vi "Autonomous Independent.vi"   [LabVIEW 2013]
doc: "This VI is called when autonomous begins, and will automatically be terminated when autonomous ends. You can carry out timed or sensor driven robot movement independently without needing to return to the caller."
uses:
  <vilib>/Rock Robotics/WPI/Solenoid/WPI_SolenoidValue.ctl
  Robot Global Data.vi
  <vilib>/Rock Robotics/WPI/RobotDrive/WPI_RobotDriveGetSetRefNum.vi
  <vilib>/Rock Robotics/WPI/RobotDrive/WPI_RobotDriveArcadeDrive_Standard(NoSaturation).vi
  <vilib>/Rock Robotics/WPI/Solenoid/Deprecated/WPI_SolenoidGetBool.vi
  <vilib>/Rock Robotics/WPI/Solenoid/WPI_SolenoidSetEnum.vi
  <vilib>/Rock Robotics/WPI/Joystick/WPI_JoystickGetSetRefNum.vi
panel:
  # "Be sure to right-click and choose Data Operations>>Make Current Value default if you want to save the array values with the VI"
types:
  T1 = typedef "WPI_SolenoidDevRef.ctl" = cluster{"DevStatus":errorcluster, "Solenoid Module":T2, "Forward Solenoid Channel":T3, "Reverse Solenoid Channel":T3}
  T2 = typedef "FPGA_TypedefSolenoidModule.ctl" = enum16{"Solenoid Module 1", "Solenoid Module 2"}
  T3 = typedef "WPI_SolenoidChannel.ctl" = enum8{"Solenoid 1", "Solenoid 2", "Solenoid 3", "Solenoid 4", "Solenoid 5", "Solenoid 6", "Solenoid 7", "Solenoid 8", "Invalid"}
  T4 = typedef "WPI_MotorControlDeviceRef.ctl" = cluster{"DeviceStatus":errorcluster, "Type":enum16{"PWM", "CAN"}, "PWM":cluster{"Digital Module":T5, "PWM Channel":T6, "DeadBand":T7}, "CAN":cluster{"Device Number":u8, "Control Mode":T8, "Semaphore":T9, "Max Vout":dbl}, "Invert":bool, "TransformRef":T10, "InvTransformRef":T10}
  T5 = typedef "FPGA_TypedefDigitalModule.ctl" = enum16{"Digital Module 1", "Digital Module 2"}
  T6 = typedef "FPGA_DIOPWMChannel.ctl" = enum8{"PWM 1", "PWM 2", "PWM 3", "PWM 4", "PWM 5", "PWM 6", "PWM 7", "PWM 8", "PWM 9", "PWM 10", "Invalid"}
  T7 = typedef "WPI_PWMDeadband.ctl" = cluster{"Name":string, "maxPositivePwm":i32, "minPositivePwm":i32, "centerPwm":i32, "maxNegativePwm":i32, "minNegativePwm":i32, "angularRange":u16}
  T8 = typedef "WPI_CANJaguar_ControlMode.ctl" = enum8{"Percent VBus", "Current", "Speed", "Position", "Voltage"}
  T9 = typedef "Semaphore RefNum" = refnum<k1>
  T10 = typedef "WPI_PWMTransform_ConPane.ctl" = refnum<vi>
  T11 = typedef "WPI_RobotDriveDevRef.ctl" = cluster{"DevStatus":errorcluster, "Motors[]":T4[], "Square Inputs":bool, "Max Output":dbl, "Isochronous":bool}
  T12 = typedef "WPI_JoystickDevRef.ctl" = cluster{"Device":T13}
  T13 = typedef "WPI_JoystickDeviceEnum.ctl" = enum16{"USB 1", "USB 2", "USB 3", "USB 4", "Kinect 1", "Kinect 2"}
  T14 = typedef "WPI_SolenoidValue.ctl" = enum16{"Off", "On", "Forward", "Reverse"}
  T15 = cluster{"axis 1 (x)":dbl, "axis 2 (y)":dbl, "axis 3 (throttle)":dbl, "axis 4":dbl, "axis 5":dbl, "axis 6":dbl}
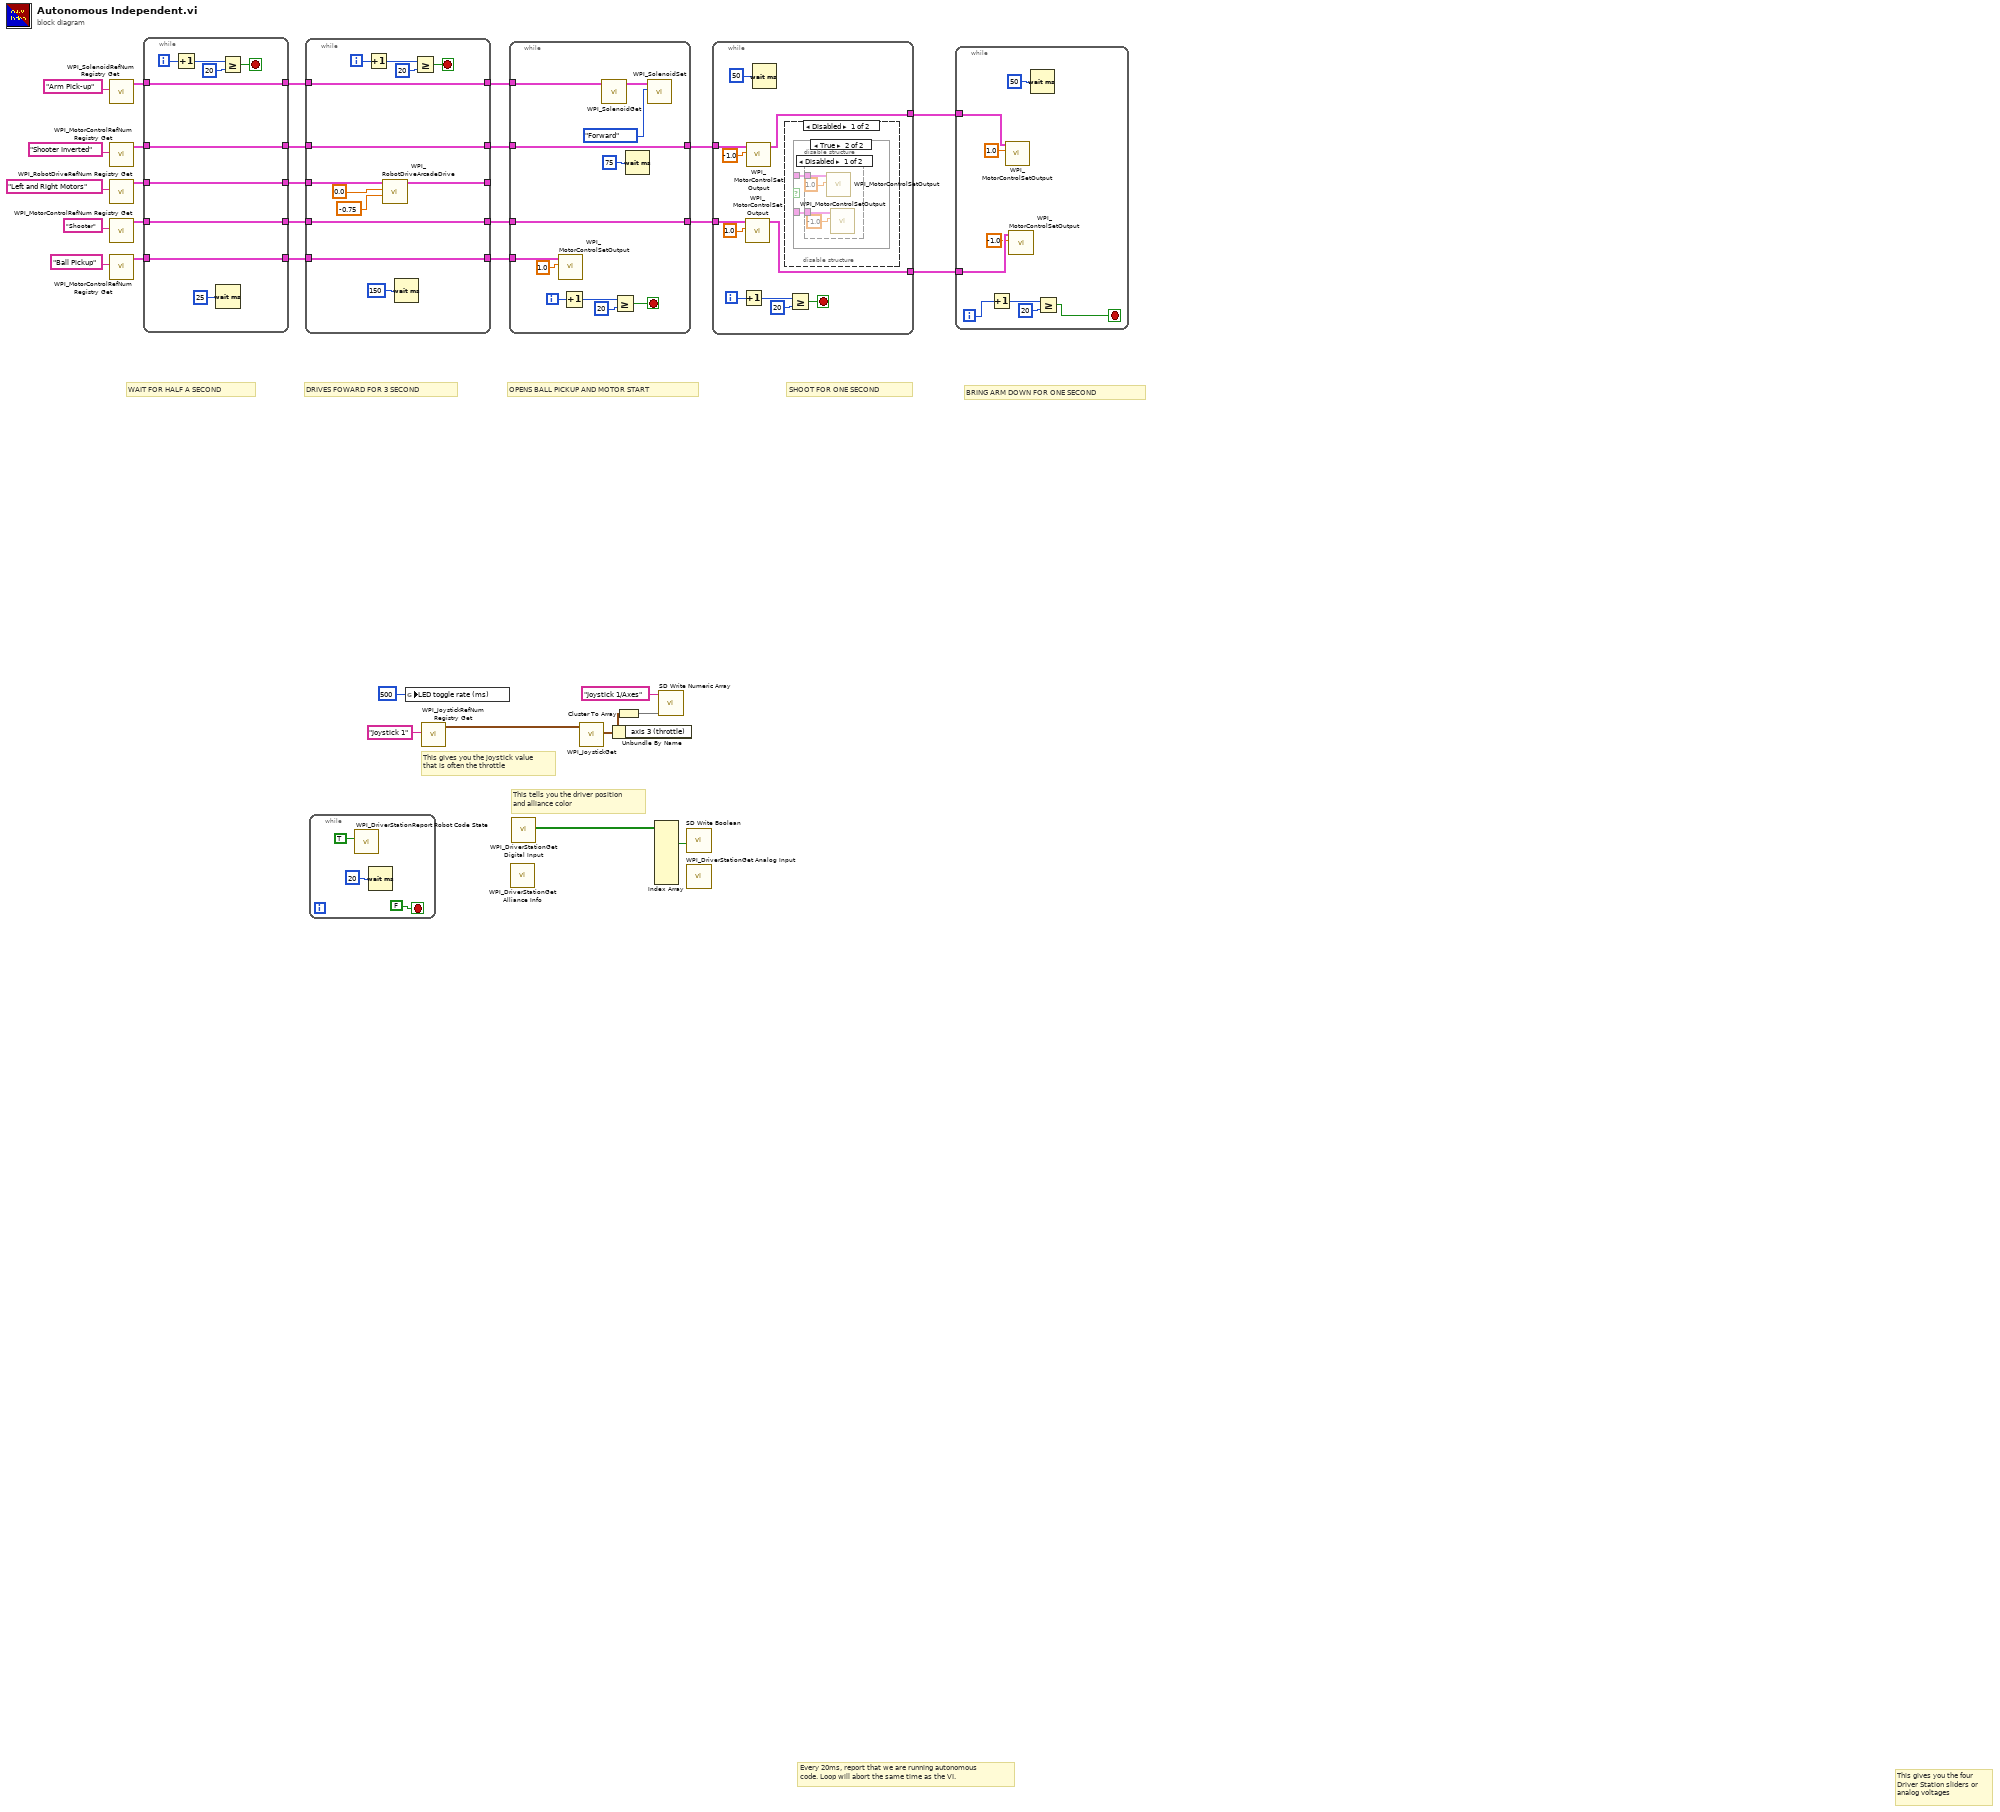
[diagram p0: block diagram]
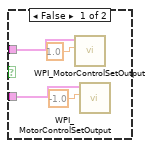
[diagram p2: hidden frame]
diagram:
  # "BRING ARM DOWN FOR ONE SECOND"
  # "WAIT FOR HALF A SECOND"
  # "SHOOT FOR ONE SECOND"
  # "OPENS BALL PICKUP AND MOTOR START"
  # "DRIVES FOWARD FOR 3 SECOND"
  # "Every 20ms, report that we are running autonomous\ncode. Loop will abort the same time as the VI."
  # "This gives you the joystick value\nthat is often the throttle"
  # "This tells you the driver position\nand alliance color"
  # "This gives you the four\nDriver Station sliders or\nanalog voltages"
  n1 = call <vilib>:"WPI_SolenoidRefNum Registry Get.vi"("refnum name"="Arm Pick-up") -> ("SolenoidDevRef"=w21:T1)  [unwired: 9 in, 1 out]
  n2 = call <vilib>:"WPI_MotorControlRefNum Registry Get.vi"("refnum name"="Shooter Inverted") -> ("MotorControlDevRef"=w17:T4)  [unwired: 9 in, 1 out]
  n3 = call <vilib>:"WPI_RobotDriveRefNum Registry Get.vi"("refnum name"="Left and Right Motors") -> ("RobotDriveDevRef"=w20:T11)  [unwired: 9 in, 1 out]
  n4 = call <vilib>:"WPI_MotorControlRefNum Registry Get.vi"("refnum name"="Shooter") -> ("MotorControlDevRef"=w16:T4)  [unwired: 9 in, 1 out]
  n5 = call <vilib>:"WPI_MotorControlRefNum Registry Get.vi"("refnum name"="Ball Pickup") -> ("MotorControlDevRef"=w14:T4)  [unwired: 9 in, 1 out]
  n6 = while {
    tunnel: w21 -> [w33]
    tunnel: [w41] -> w13
    tunnel: w20 -> [w41]
    tunnel: w17 -> [w35]
    tunnel: [w35] -> w11
    tunnel: w16 -> [w34]
    tunnel: [w34] -> w12
    tunnel: w14 -> [w32]
    tunnel: [w33] -> w6
    tunnel: [w32] -> w4
    i -> [w38]
    stop <- w37 stop-if-true
    n7 = Increment(x=w38) -> (x+1=w39:i32)
    n8 = Wait (ms)(milliseconds to wait=u32 25) -> ()  [unwired: 1 out]
    n9 = Greater Or Equal?(x=w39, y=20) -> (x >= y?=w37:bool)
  }
  n10 = while {
    tunnel: w13 -> [w54]
    tunnel: [w47] -> _
    tunnel: w11 -> [w45]
    tunnel: [w45] -> w9
    tunnel: w12 -> [w44]
    tunnel: [w44] -> w7
    tunnel: w6 -> [w43]
    tunnel: [w43] -> w5
    tunnel: [w42] -> w3
    tunnel: w4 -> [w42]
    i -> [w52]
    stop <- w49 stop-if-true
    n11 = Increment(x=w52) -> (x+1=w51:i32)
    n12 = call-poly <vilib>:"WPI_RobotDriveArcadeDrive.vi"("Y axis value"=-0.75, "X axis value"=0.0, "RobotDriveDevRef"=w54) -> ("RobotDriveDevRef"=w47:T11)  [unwired: 6 in, 2 out]
    n13 = Wait (ms)(milliseconds to wait=u32 150) -> ()  [unwired: 1 out]
    n14 = Greater Or Equal?(x=w51, y=20) -> (x >= y?=w49:bool)
  }
  n15 = while {
    stop <- FALSE stop-if-true
    n16 = call <vilib>:"WPI_DriverStationReport Robot Code State.vi"("Autonomous"=TRUE) -> ()  [unwired: 10 in, 1 out]
    n17 = Wait (ms)(milliseconds to wait=u32 20) -> ()  [unwired: 1 out]
  }
  n18 = global write "Robot Global Data.vi" "LED toggle rate (ms)"(u32 500 ("LED ms toggle rate")) -> ()
  n19 = call <vilib>:"WPI_JoystickRefNum Registry Get.vi"("refnum name"="Joystick 1") -> ("JoystickDevRef"=w29:T12)  [unwired: 1 in, 9 out]
  n20 = while {
    tunnel: [w69] -> w10
    tunnel: w9 -> [w69]
    tunnel: [w68] -> w8
    tunnel: w7 -> [w68]
    tunnel: w5 -> [w60]
    tunnel: w3 -> [w58]
    i -> [w66]
    stop <- w64 stop-if-true
    n21 = call <vilib>:"WPI_MotorControlSetOutput.vi"("Output"=1.0, "MotorControlDevRef"=w58) -> ()  [unwired: 7 in, 3 out]
    n22 = Increment(x=w66) -> (x+1=w67:i32)
    n23 = call-poly <vilib>:"WPI_SolenoidGet.vi"("SolenoidDevRef"=w60) -> ("SolenoidDevRef"=w61:T1)  [unwired: 8 in, 2 out]
    n24 = Greater Or Equal?(x=w67, y=20) -> (x >= y?=w64:bool)
    n25 = Wait (ms)(milliseconds to wait=u32 75) -> ()  [unwired: 1 out]
    n26 = call-poly <vilib>:"WPI_SolenoidSet.vi"("Value"=WPI_SolenoidValue."Forward", "SolenoidDevRef"=w61) -> ()  [unwired: 8 in, 2 out]
  }
  n27 = call <vilib>:"WPI_DriverStationGet Alliance Info.vi"() -> ()  [unwired: 12 out]
  n28 = call <vilib>:"WPI_DriverStationGet Digital Input.vi"() -> ("Driver Station Digital Input (1-8)"=w31:bool[])  [unwired: 11 out]
  n29 = call <vilib>:"WPI_JoystickGet.vi"("JoystickDevRef"=w29) -> ("Axes"=w26:T15)  [unwired: 1 in, 5 out]
  n30 = Unbundle By Name(w26) -> ()  [unwired: 1 out]
  n31 = Cluster To Array(cluster=w26) -> (array=w27:dbl[])
  n32 = Index Array(array=w31) -> (element #2=w24:bool)  [unwired: 8 in, 7 out]
  n33 = call <vilib>:"SD Write Numeric Array.vi"("Numeric Array"=w27, "Name"="Joystick 1/Axes") -> ()  [unwired: 8 in, 2 out]
  n34 = call <vilib>:"SD Write Boolean.vi"("Boolean"=w24) -> ()  [unwired: 9 in, 2 out]
  n35 = call <vilib>:"WPI_DriverStationGet Analog Input.vi"() -> ()  [unwired: 12 out]
  n36 = while {
    tunnel: w10 -> [w75]
    tunnel: w8 -> [w74]
    tunnel: [w71] -> w2
    tunnel: [w70] -> w1
    i -> [w78]
    stop <- w77 stop-if-true
    n37 = Increment(x=w78) -> (x+1=w80:i32)
    n38 = call <vilib>:"WPI_MotorControlSetOutput.vi"("Output"=1.0, "MotorControlDevRef"=w74) -> ("MotorControlDevRef"=w70:T4)  [unwired: 7 in, 2 out]
    n39 = call <vilib>:"WPI_MotorControlSetOutput.vi"("Output"=-1.0, "MotorControlDevRef"=w75) -> ("MotorControlDevRef"=w71:T4)  [unwired: 7 in, 2 out]
    n40 = Wait (ms)(milliseconds to wait=u32 50) -> ()  [unwired: 1 out]
    n41 = disable-structure shown="Disabled" {
      frame Disabled {
        n42 = case shown="True" {
          selector: _ -> [_ _]
          tunnel: _ -> [w82 w86]
          tunnel: _ -> [w81 w85]
          frame False {
            n43 = call <vilib>:"WPI_MotorControlSetOutput.vi"("Output"=1.0, "MotorControlDevRef"=w82) -> ()  [unwired: 7 in, 3 out]
            n44 = call <vilib>:"WPI_MotorControlSetOutput.vi"("Output"=-1.0, "MotorControlDevRef"=w81) -> ()  [unwired: 7 in, 3 out]
          }
          frame True {
            n45 = disable-structure shown="Disabled" {
              disable-tunnel: w86 -> [w90 _]
              disable-tunnel: w85 -> [w87 _]
              frame Disabled {
                n46 = call <vilib>:"WPI_MotorControlSetOutput.vi"("Output"=1.0, "MotorControlDevRef"=w90) -> ()  [unwired: 7 in, 3 out]
                n47 = call <vilib>:"WPI_MotorControlSetOutput.vi"("Output"=-1.0, "MotorControlDevRef"=w87) -> ()  [unwired: 7 in, 3 out]
              }
              frame Enabled {
              }
            }
          }
        }
      }
      frame Enabled {
      }
    }
    n48 = Greater Or Equal?(x=w80, y=20) -> (x >= y?=w77:bool)
  }
  n49 = while {
    tunnel: w2 -> [w99]
    tunnel: w1 -> [w98]
    i -> [w95]
    stop <- w94 stop-if-true
    n50 = Increment(x=w95) -> (x+1=w96:i32)
    n51 = call <vilib>:"WPI_MotorControlSetOutput.vi"("Output"=1.0, "MotorControlDevRef"=w99) -> ()  [unwired: 7 in, 3 out]
    n52 = call <vilib>:"WPI_MotorControlSetOutput.vi"("Output"=-1.0, "MotorControlDevRef"=w98) -> ()  [unwired: 7 in, 3 out]
    n53 = Wait (ms)(milliseconds to wait=u32 50) -> ()  [unwired: 1 out]
    n54 = Greater Or Equal?(x=w96, y=20) -> (x >= y?=w94:bool)
  }
